vi "PCO_SetAcquireModeEx.vi"(8 "error in (no error)":errorcluster {"code" format="%x"}, 9 "dwNumberImages":u32, 10 "wAcquMode":u16(ring) items=["auto", "external", "external modulate", "", "sequence trigger"], 11 "ph":u64) -> (0 "error out":errorcluster {"code" format="%x"}, 2 "ErrorMessage":i32 format="%x", 3 "ph out":u64)   [LabVIEW 2019, in "SDK.lvlib" / "RecordingControl.lvlib"]
doc: "<b>Description:</b>\nThis function sets the acquire mode of the camera. Acquire mode can be either [auto], [external], [external modulate] or [sequence trigger]. This function is an extended version of the PCO_SetAcquireMode function with an additional parameter dwNumberImages, which is needed for the [sequence trigger] mode.\n\n<b>Supported camera type:</b>\npco.edge\n\n<b>Descriptor dependency:</b>\ndwGeneralCapsDESC1: NO_ACQUIREMODE,EXT_ACQUIRE"
uses:
  RecordingControl.lvlib
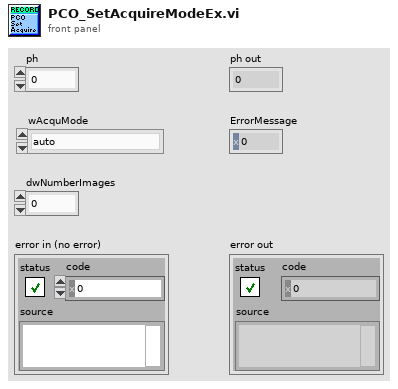
[diagram p1: front panel]
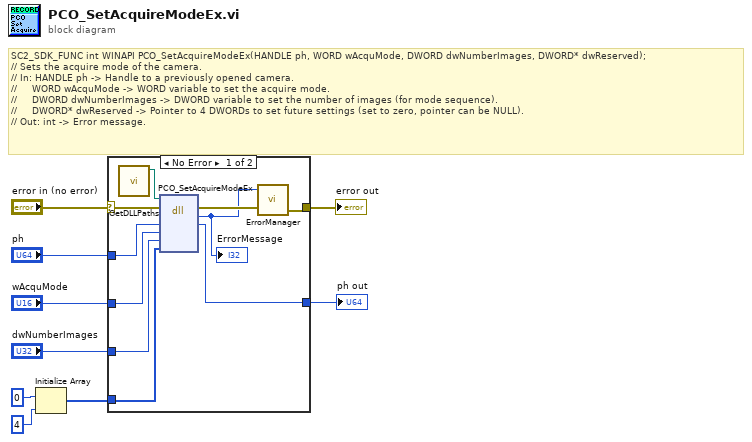
[diagram p0: block diagram]
diagram:
  # "SC2_SDK_FUNC int WINAPI PCO_SetAcquireModeEx(HANDLE ph, WORD wAcquMode, DWORD dwNumberImages, DWORD* dwReserved);\n// Sets the acquire mode of the camera.\n// In: HANDLE ph -> Handle to a previously opened camera.\n//     WORD wAcquMode -> WORD variable to set the acquire mode.\n//     DWORD dwNumberImages -> DWORD variable to set the number of images (for mode sequence).\n//     DWORD* dwReserved -> Pointer to 4 DWORDs to set future settings (set to zero, pointer can be NULL).\n// Out: int -> Error message."
  n1 = Initialize Array(u32 0, 4 ("dimension size")) -> (w2:u32[])
  n2 = case shown="No Error" "error in (no error)" {
    selector: "error in (no error)" -> [w14 w21]
    tunnel: "ph" -> [w19 w20]
    tunnel: [w18 w20] -> w8
    tunnel: "wAcquMode" -> [w17 _]
    tunnel: "dwNumberImages" -> [w16 _]
    tunnel: [w12 w21] -> w5
    tunnel: w2 -> [w15 _]
    frame No Error {
      n3 = call "GetDLLPaths.vi"() -> ("SC2_Cam_Path"=w10:path)  [unwired: 9 in, 2 out]
      n4 = dll-call lib="?" fn="PCO_SetAcquireModeEx"(path in=w10, error in=w14, "ph"=w19, "wAcquMode"=w17, "dwNumberImages"=w16, "dwReserved"=w15) -> (error out=w13:errorcluster, "return type"=w11:i32, "ph"=w18:u64)  [unwired: 4 in, 1 out]
      "ErrorMessage" <- w11
      n5 = call "ErrorManager.vi"("error in (no error)"=w13, "error code"=w11) -> ("error out"=w12:errorcluster)  [unwired: 3 in]
    }
    frame Error {
    }
  }
  "ph out" <- w8
  "error out" <- w5
